vi "MGI RWA String To Anything.vi"(5 "Use Supplied":bool, 7 "Format String (%#_13g)":string="%#_13g", 8 "Error In":errorcluster, 9 "String":string, 10 "Type of Anything":variant, 11 "Read/Write Options":T1={"TS Fmt"="", "Int Fmt"="", "Delimiter"=","}) -> (0 "Error Out":errorcluster, 2 "Read Failures":string, 3 "Variant":variant)   [LabVIEW 2016]
doc: "Parse the specified String to populate the specified datatype. If string doesn't contain a field defined by datatype, then that field is set based on \"Use Supplied\". If \"Use Supplied\" is true, then the field is left as is, otherwise the field is set to default value.\n\nAuthored by Robert C. Mortensen\nsupport@mooregoodideas.com\nwww.mooregoodideas.com\n\nCopyright (c) 2010, Moore Good Ideas, Inc.\n\nAll rights reserved.\n\nRedistribution and use in source and binary forms, with or without modification, are permitted provided that the following conditions are met:\n\n * Redistributions of source code must retain the above copyright notice, this list of conditions and the following disclaimer.\n * Redistributions in binary form must reproduce the above copyright notice, this list of conditions and the following disclaimer in the documentation and/or other materials provided with the distribution.\n * Neither the name of Moore Good Ideas, Inc. nor the names of its contributors may be used to endorse or promote products derived from this software without specific prior written permission.\n\nTHIS SOFTWARE IS PROVIDED BY THE COPYRIGHT HOLDERS AND CONTRIBUTORS \"AS IS\" AND ANY EXPRESS OR IMPLIED WARRANTIES, INCLUDING, BUT NOT LIMITED TO, THE IMPLIED WARRANTIES OF MERCHANTABILITY AND FITNESS FOR A PARTICULAR PURPOSE ARE DISCLAIMED. IN NO EVENT SHALL THE COPYRIGHT OWNER OR CONTRIBUTORS BE LIABLE FOR ANY DIRECT, INDIRECT, INCIDENTAL, SPECIAL, EXEMPLARY, OR CONSEQUENTIAL DAMAGES (INCLUDING, BUT NOT LIMITED TO, PROCUREMENT OF SUBSTITUTE GOODS OR SERVICES; LOSS OF USE, DATA, OR PROFITS; OR BUSINESS INTERRUPTION) HOWEVER CAUSED AND ON ANY THEORY OF LIABILITY, WHETHER IN CONTRACT, STRICT LIABILITY, OR TORT (INCLUDING NEGLIGENCE OR OTHERWISE) ARISING IN ANY WAY OUT OF THE USE OF THIS SOFTWARE, EVEN IF ADVISED OF THE POSSIBILITY OF SUCH DAMAGE."
uses:
  <userlib>/_MGI/Read Write Anything/MGI RWA Options Cluster.ctl
  <userlib>/_MGI/Read Write Anything/MGI RWA Convertion Direction Enum.ctl
  <vilib>/Utility/VariantDataType/Type.ctl
  <userlib>/_MGI/String/MGI Scan From String/MGI Scan From String (CSG).vi
  <userlib>/_MGI/String/MGI Scan From String/MGI Scan From String (CDB).vi
  <userlib>/_MGI/String/MGI Scan From String/MGI Scan From String (CXT).vi
  <vilib>/Utility/VariantDataType/VariantType.lvlib
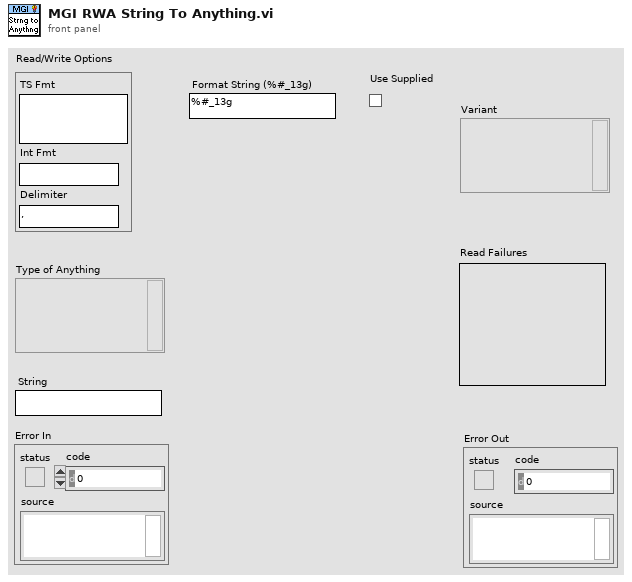
[diagram p1: front panel]
types:
  T1 = typedef "MGI RWA Options Cluster.ctl" = cluster{"TS Fmt":string, "Int Fmt":string, "Delimiter":string}
  T2 = typedef "MGI RWA Convertion Direction Enum.ctl" = enum16{"String->Anything", "Anything->String"}
  T3 = typedef "MGI RWA Tag Lookup Cluster.ctl" = cluster{"StrToSpecifiedText":variant, "Specified Data":variant, "Float Fmt":string, "Major Vers":i32, "Options":T1}
  T4 = typedef "VariantType.lvlib/Type.ctl" = enum8{"Invalid Type", "Void", "I8", "I16", "I32", "I64", "U8", "U16", "U32", "U64", "Single Float", "Double Float", "Extended Float", "Single Complex", "Double Complex", "Extended Complex", "Enum U8", "Enum U16", "Enum U32", "Enum U64", "Single Float With Unit", "Double Float With Unit", "Extended Float With Unit", "Single Complex with Unit", "Double Complex with Unit", "Extended Complex with Unit", "Boolean", "String", "Path", "Picture", "Tag", "Array", "Cluster", "Variant", "LV Variant", "Waveform", "Timestamp", "Digital Waveform", "Digital Data", "ExpressData", "Refnum", "External Data", "VI", "Poly VI", "LabVIEW Class Instance", "Fixed Point"}
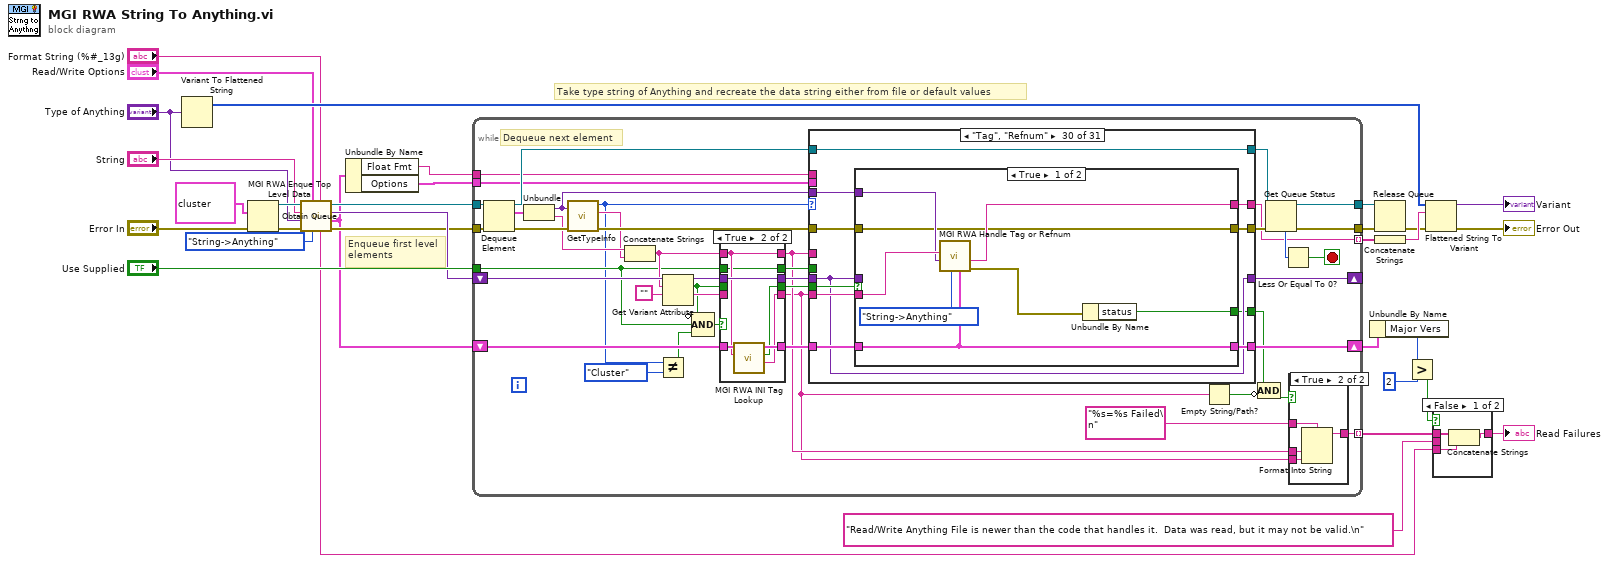
[diagram p0: block diagram]
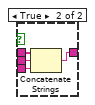
[diagram p2: hidden frame]
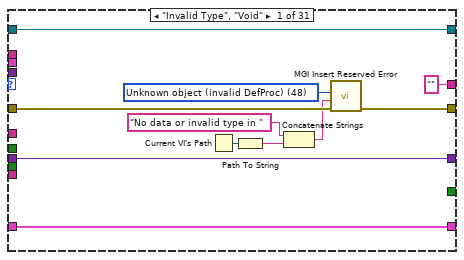
[diagram p5: hidden frame]
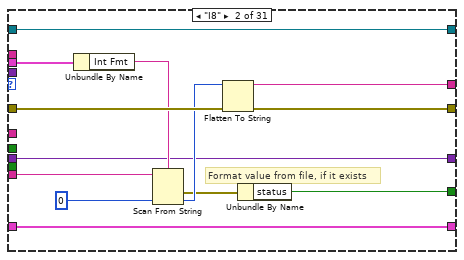
[diagram p6: hidden frame]
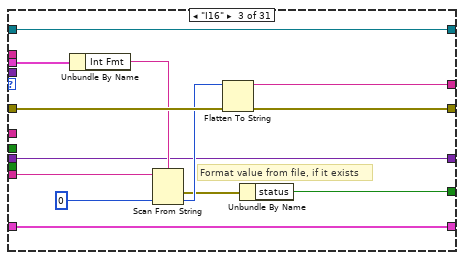
[diagram p7: hidden frame]
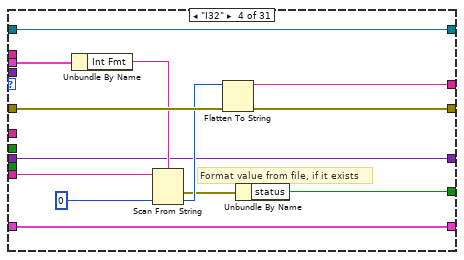
[diagram p8: hidden frame]
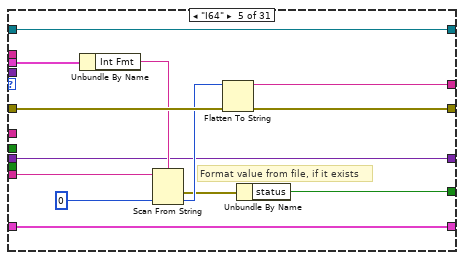
[diagram p9: hidden frame]
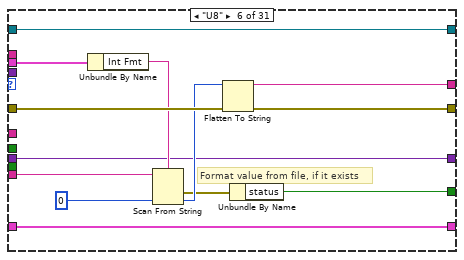
[diagram p10: hidden frame]
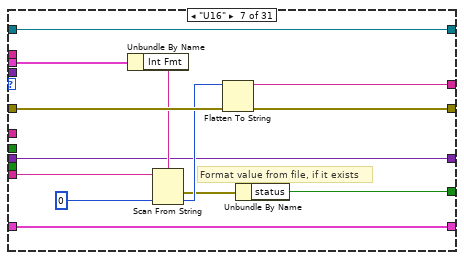
[diagram p11: hidden frame]
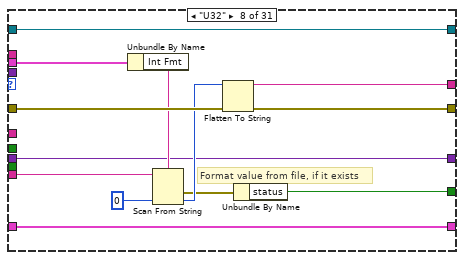
[diagram p12: hidden frame]
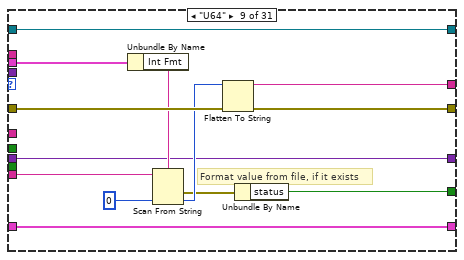
[diagram p13: hidden frame]
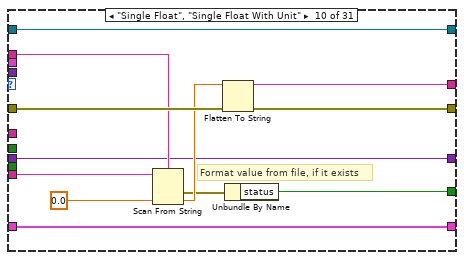
[diagram p14: hidden frame]
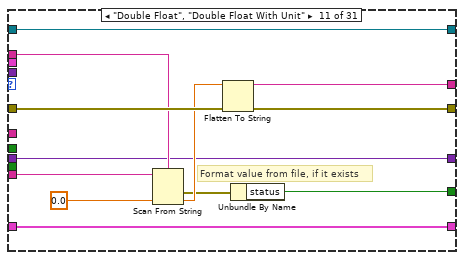
[diagram p15: hidden frame]
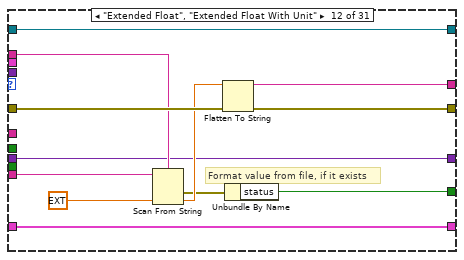
[diagram p16: hidden frame]
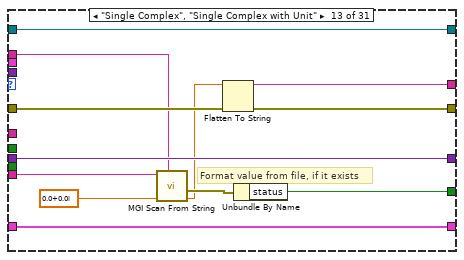
[diagram p17: hidden frame]
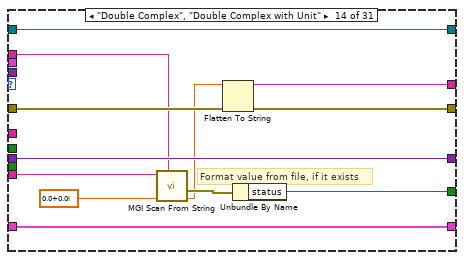
[diagram p18: hidden frame]
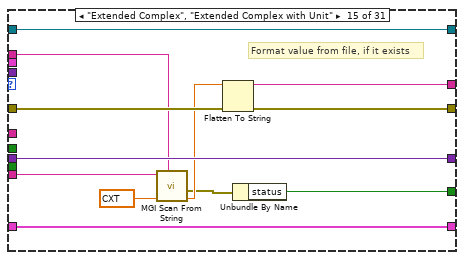
[diagram p19: hidden frame]
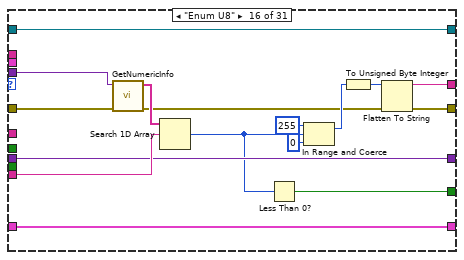
[diagram p20: hidden frame]
diagram:
  # "Enqueue first level\nelements"
  # "Take type string of Anything and recreate the data string either from file or default values"
  n1 = Variant To Flattened String(Variant="Type of Anything") -> (1:w25:i16[])  [unwired: 1 out]
  n2 = Obtain Queue(element data type=cluster{"Variant":variant, "Name":string} {"Variant"=variant, "Name"=""}, error in (no error)="Error In") -> (queue out=w23:refnum<queue>, error out=w17:errorcluster)  [unwired: 3 in, 1 out]
  n3 = call <userlib>:"MGI RWA Enque Top Level Data.vi"("Format String (%#_13g)"="Format String (%#_13g)", "Conversion"=MGI_RWA_Convertion_Direction_Enum."String->Anything", "Read/Write Options"="Read/Write Options", "Error In"=w17, "Anything"="Type of Anything", "Read String"="String", "Data Queue In"=w23) -> ("Error Out"=w20:errorcluster, "Read State"=w15:T3, "Tag to String"=w22:variant, "Data Queue Our"=w21:refnum<queue>, "Warnings"=w1:string)
  n4 = Unbundle By Name(w15) -> ("Float Fmt"=w13:string, "Options"=w11:T1)
  n5 = while {
    tunnel: w20 -> [w74]
    tunnel: [w40] -> w28
    tunnel: [w61] -> w27 mode=indexing
    tunnel: w21 -> [w71]
    tunnel: [w66] -> w30
    tunnel: w11 -> [w42]
    tunnel: w13 -> [w41]
    shift-right: [w47] -> w10
    shift-left: w15 -> [w51]
    shift-right: [w46] -> _
    shift-left: w22 -> [w59]
    tunnel: "Use Supplied" -> [w50]
    tunnel: [w33] -> w6 mode=indexing
    stop <- w67 stop-if-true
    # "Dequeue next element"
    n6 = Dequeue Element(queue=w71, error in (no error)=w74) -> (queue out=w72:refnum<queue>, element=w65:cluster{"Variant":variant, "Name":string}, error out=w73:errorcluster)  [unwired: 1 in, 1 out]
    n7 = Unbundle(w65) -> ("Variant"=w63:variant, "Name"=w64:string)
    n8 = call <vilib>:"GetTypeInfo.vi"("error in (no error)"=w73, "Variant"=w63) -> ("error out"=w75:errorcluster, "Name"=w62:string, "Type Enum"=w45:T4)  [unwired: 5 in, 2 out]
    n9 = Concatenate Strings(w64, w62) -> (w55:string)
    n10 = Not Equal?(x=w45, y=Type."Cluster") -> (x != y?=w44:bool)
    n11 = Get Variant Attribute(Variant=w59, name=w55, default value (empty Variant)="") -> (duplicate Variant=w54:variant, found=w57:bool, value=w58:string)  [unwired: 1 in, 1 out]
    n12 = Compound Arithmetic op=AND(invert w57, w50, w44) -> (w56:bool)
    n13 = case shown="True" w56 {
      tunnel: w58 -> [w82 _]
      tunnel: w57 -> [w83 _]
      tunnel: w55 -> [w84 w87]
      tunnel: w54 -> [w85 w91]
      tunnel: [w85 w91] -> w53
      tunnel: [w84 w87] -> w36
      tunnel: [w83 w89] -> w52
      tunnel: [w82 w88] -> w35
      tunnel: w51 -> [w81 w92]
      tunnel: [w81 w90] -> w48
      tunnel: w50 -> [w80 w86]
      tunnel: [w80 w86] -> w49
      frame False {
      }
      frame True {
        n14 = call <userlib>:"MGI RWA INI Tag Lookup.vi"("String"=w87, "State In"=w92) -> ("INI Text"=w88:string, "Text Found?"=w89:bool, "State Out"=w90:T3)  [unwired: 7 in]
      }
    }
    n15 = case shown="\"Tag\", \"Refnum\"" w45 {
      tunnel: [w97 w116 w129 w142 w155 w168 w181 w194 w207 w219 w231 w243 w255 w267 w279 w295 w311 w327 w343 w353 w361 w369 w377 w398 w426 w459 w505 w533 w565 w580 w601] -> w70
      tunnel: w75 -> [w98 w115 w128 w141 w154 w167 w180 w193 w206 w218 w230 w242 w254 w266 w278 w294 w310 w326 w342 w352 w360 w368 w383 w397 w425 w458 w504 w532 w568 w579 w600]
      tunnel: w36 -> [_ _ _ _ _ _ _ _ _ _ _ _ _ _ _ _ _ _ _ _ _ _ w370 _ _ _ _ _ w562 _ _]
      tunnel: ["" ("data string") w114 w127 w140 w153 w166 w179 w192 w205 w217 w229 w241 w253 w265 w277 w293 w309 w325 w341 w351 w359 w367 "" w396 w424 w457 w503 w531 w557 w578 w599] -> w61
      tunnel: w63 -> [_ _ _ _ _ _ _ _ _ _ _ _ _ _ _ w292 w308 w324 w340 _ _ _ w382 _ _ _ _ _ w567 w571 _]
      tunnel: w72 -> [w99 w113 w126 w139 w152 w165 w178 w191 w204 w216 w228 w240 w252 w264 w276 w291 w307 w323 w339 w350 w358 w366 w378 w395 w423 w456 w502 w530 w569 w577 w598]
      tunnel: [w99 w113 w126 w139 w152 w165 w178 w191 w204 w216 w228 w240 w252 w264 w276 w291 w307 w323 w339 w350 w358 w366 w376 w395 w423 w456 w502 w530 w564 w577 w598] -> w69
      tunnel: w53 -> [w94 w108 w121 w134 w147 w160 w173 w186 w200 w211 w223 w235 w251 w263 w275 w283 w299 w316 w331 w345 w356 w363 w372 w393 w420 w449 w499 w527 w561 w572 w595]
      tunnel: w42 -> [_ w106 w119 w132 w145 w158 w171 w184 w197 _ _ _ _ _ _ _ _ _ _ _ _ _ _ _ _ _ _ _ w556 _ _]
      tunnel: w41 -> [_ _ _ _ _ _ _ _ _ w213 w225 w237 w246 w259 w270 _ _ _ _ _ _ _ _ _ _ _ _ _ w555 _ _]
      tunnel: [w94 w108 w121 w134 w147 w160 w173 w186 w200 w211 w223 w235 w251 w263 w275 w283 w299 w316 w331 w345 w356 w363 w372 w393 w420 w449 w499 w527 w558 w572 w595] -> w46
      tunnel: w35 -> [_ w109 w122 w135 w148 w161 w174 w187 w199 w212 w224 w236 w245 w256 w271 w284 w300 w317 w332 w346 w357 w364 _ w394 w422 w450 w500 w528 w566 w575 w596]
      tunnel: w52 -> [_ _ _ _ _ _ _ _ _ _ _ _ _ _ _ _ _ _ _ _ _ _ _ w392 w421 w451 w501 w529 _ w576 w597]
      tunnel: w49 -> [_ _ _ _ _ _ _ _ _ _ _ _ _ _ _ _ _ _ _ _ _ _ _ _ _ _ _ _ w563 _ _]
      tunnel: w48 -> [w93 w107 w120 w133 w146 w159 w172 w185 w198 w210 w222 w234 w250 w262 w274 w282 w298 w315 w330 w344 w355 w362 w371 w391 w419 w448 w498 w526 w560 w574 w594]
      tunnel: [w93 w107 w120 w133 w146 w159 w172 w185 w198 w210 w222 w234 w250 w262 w274 w282 w298 w315 w330 w344 w355 w362 w371 w391 w419 w448 w498 w526 w559 w573 w594] -> w47
      tunnel: [_ w104 w117 w130 w143 w156 w169 w182 w195 w208 w220 w232 w249 w261 w273 w280 w296 w312 w328 _ _ _ _ _ _ w447 _ _ w554 w570 _] -> w39
      frame "Invalid Type", "Void" {
        w95 = u16 48 items=["No error", "Argument error", "Memory is full", "Out of zone", "End of file", "File already open", "Generic file I/O error", "File not found", "File permission error", "Disk is full", "Duplicate path", "Too many files open", "System feature not enabled", "Resource file not found", "Cannot add resource", "Resource not found", "Image not found", "Image memory error", "Pen does not exist", "Config type invalid", "Config token not found", "Config parse error", "Config memory error", "Bad external code format", "Bad external code offset", "External code not present", "Null window", "Destroy window error", "Null menu", "Print aborted", "Bad print record", "Print driver error", "Windows error during printing", "Memory error during printing", "Print dialog error", "Generic print error", "Invalid device refnum", "Device not found", "Device parameter error", "Device unit error", "Cannot open device", "Device call aborted", "Generic error", "Cancelled by user", "Object ID too low", "Object ID too high", "Object not in heap", "Unknown heap", "Unknown object (invalid DefProc)", "Unknown object (DefProc not in table)", "Message out of range", "Invalid (null) method", "Unknown message", "Manager call not supported", "Bad address", "Network operation in progress", "Network operation timed out", "Connection is busy", "Network attribute not supported", "Network error", "Address in use", "System out of memory", "Connection aborted", "Connection refused", "Not connected", "Already connected", "Connection closed", "Initialization error (interapplication manager)", "Bad occurrence", "Wait on unbound occurrence handler", "Occurrence queue overflow", "Datalog type conflict", "Unused", "Unrecognized type (interapplication manager)", "Memory corrupt", "Failed to make temporary DLL", "Old CIN version", "Drag socket not found", "Failed to load drop-object", "Failed to register OLE object", "Failed to release OLE object", "Format specifier type mismatch", "Unknown format specifier", "Too few format specifiers", "Too many format specifiers", "Scan failed", "Newer CIN version", "OLE Convert", "Runtime menu error", "Password tampered", "Unknown error code"] ("Reserved Error Code")
        n16 = Current VI's Path() -> (path=w101:path)
        n17 = Path To String(path=w101) -> (string=w100:string)
        n18 = Concatenate Strings("No data or invalid type in " ("string"), w100) -> (w96:string)
        n19 = call <userlib>:"MGI Insert Reserved Error.vi"("Error In"=w98, "Error Description"=w96, "Reserved Error Code (Generic error)"=w95) -> ("Error Out"=w97:errorcluster)  [unwired: 8 in]
      }
      frame "I8" {
        # "Format value from file, if it exists"
        n20 = Unbundle By Name(w106) -> ("Int Fmt"=w111:string)
        n21 = Scan From String(format string=w111, input string=w109, default 1=i8 0 ("default (0 I32)")) -> (error out=w105:errorcluster, output 1=w110:i8)  [unwired: 2 in, 2 out]
        n22 = Flatten To String(anything=w110, error in (no error)=w115) -> (data string=w114:string, error out=w116:errorcluster)  [unwired: 2 in, 1 out]
        n23 = Unbundle By Name(w105) -> ("status"=w104:bool)
      }
      frame "I16" {
        # "Format value from file, if it exists"
        n24 = Unbundle By Name(w119) -> ("Int Fmt"=w124:string)
        n25 = Scan From String(format string=w124, input string=w122, default 1=i16 0 ("default (0 I32)")) -> (error out=w118:errorcluster, output 1=w123:i16)  [unwired: 2 in, 2 out]
        n26 = Flatten To String(anything=w123, error in (no error)=w128) -> (data string=w127:string, error out=w129:errorcluster)  [unwired: 2 in, 1 out]
        n27 = Unbundle By Name(w118) -> ("status"=w117:bool)
      }
      frame "I32" {
        # "Format value from file, if it exists"
        n28 = Unbundle By Name(w132) -> ("Int Fmt"=w137:string)
        n29 = Scan From String(format string=w137, input string=w135, default 1=0 ("default (0 I32)")) -> (error out=w131:errorcluster, output 1=w136:i32)  [unwired: 2 in, 2 out]
        n30 = Flatten To String(anything=w136, error in (no error)=w141) -> (data string=w140:string, error out=w142:errorcluster)  [unwired: 2 in, 1 out]
        n31 = Unbundle By Name(w131) -> ("status"=w130:bool)
      }
      frame "I64" {
        # "Format value from file, if it exists"
        n32 = Unbundle By Name(w145) -> ("Int Fmt"=w150:string)
        n33 = Scan From String(format string=w150, input string=w148, default 1=i64 0 ("default (0 I32)")) -> (error out=w144:errorcluster, output 1=w149:i64)  [unwired: 2 in, 2 out]
        n34 = Flatten To String(anything=w149, error in (no error)=w154) -> (data string=w153:string, error out=w155:errorcluster)  [unwired: 2 in, 1 out]
        n35 = Unbundle By Name(w144) -> ("status"=w143:bool)
      }
      frame "U8" {
        # "Format value from file, if it exists"
        n36 = Unbundle By Name(w158) -> ("Int Fmt"=w163:string)
        n37 = Scan From String(format string=w163, input string=w161, default 1=u8 0 ("default (0 I32)")) -> (error out=w157:errorcluster, output 1=w162:u8)  [unwired: 2 in, 2 out]
        n38 = Flatten To String(anything=w162, error in (no error)=w167) -> (data string=w166:string, error out=w168:errorcluster)  [unwired: 2 in, 1 out]
        n39 = Unbundle By Name(w157) -> ("status"=w156:bool)
      }
      frame "U16" {
        # "Format value from file, if it exists"
        n40 = Unbundle By Name(w171) -> ("Int Fmt"=w176:string)
        n41 = Scan From String(format string=w176, input string=w174, default 1=u16 0 ("default (0 I32)")) -> (error out=w170:errorcluster, output 1=w175:u16)  [unwired: 2 in, 2 out]
        n42 = Flatten To String(anything=w175, error in (no error)=w180) -> (data string=w179:string, error out=w181:errorcluster)  [unwired: 2 in, 1 out]
        n43 = Unbundle By Name(w170) -> ("status"=w169:bool)
      }
      frame "U32" {
        # "Format value from file, if it exists"
        n44 = Unbundle By Name(w184) -> ("Int Fmt"=w189:string)
        n45 = Scan From String(format string=w189, input string=w187, default 1=u32 0 ("default (0 I32)")) -> (error out=w183:errorcluster, output 1=w188:u32)  [unwired: 2 in, 2 out]
        n46 = Flatten To String(anything=w188, error in (no error)=w193) -> (data string=w192:string, error out=w194:errorcluster)  [unwired: 2 in, 1 out]
        n47 = Unbundle By Name(w183) -> ("status"=w182:bool)
      }
      frame "U64" {
        # "Format value from file, if it exists"
        n48 = Unbundle By Name(w197) -> ("Int Fmt"=w202:string)
        n49 = Scan From String(format string=w202, input string=w199, default 1=u64 0 ("default (0 I32)")) -> (error out=w196:errorcluster, output 1=w201:u64)  [unwired: 2 in, 2 out]
        n50 = Flatten To String(anything=w201, error in (no error)=w206) -> (data string=w205:string, error out=w207:errorcluster)  [unwired: 2 in, 1 out]
        n51 = Unbundle By Name(w196) -> ("status"=w195:bool)
      }
      frame "Single Float", "Single Float With Unit" {
        # "Format value from file, if it exists"
        n52 = Scan From String(format string=w213, input string=w212, default 1=sgl 0.0 ("default (0 I32)")) -> (error out=w209:errorcluster, output 1=w214:sgl)  [unwired: 2 in, 2 out]
        n53 = Flatten To String(anything=w214, error in (no error)=w218) -> (data string=w217:string, error out=w219:errorcluster)  [unwired: 2 in, 1 out]
        n54 = Unbundle By Name(w209) -> ("status"=w208:bool)
      }
      frame "Double Float", "Double Float With Unit" {
        # "Format value from file, if it exists"
        n55 = Scan From String(format string=w225, input string=w224, default 1=0.0 ("default (0 I32)")) -> (error out=w221:errorcluster, output 1=w226:dbl)  [unwired: 2 in, 2 out]
        n56 = Flatten To String(anything=w226, error in (no error)=w230) -> (data string=w229:string, error out=w231:errorcluster)  [unwired: 2 in, 1 out]
        n57 = Unbundle By Name(w221) -> ("status"=w220:bool)
      }
      frame "Extended Float", "Extended Float With Unit" {
        # "Format value from file, if it exists"
        n58 = Scan From String(format string=w237, input string=w236, default 1=ext 0.0 ("default (0 I32)")) -> (error out=w233:errorcluster, output 1=w238:ext)  [unwired: 2 in, 2 out]
        n59 = Flatten To String(anything=w238, error in (no error)=w242) -> (data string=w241:string, error out=w243:errorcluster)  [unwired: 2 in, 1 out]
        n60 = Unbundle By Name(w233) -> ("status"=w232:bool)
      }
      frame "Single Complex", "Single Complex with Unit" {
        # "Format value from file, if it exists"
        n61 = call-poly <userlib>:"MGI Scan From String.vi"("format string"=w246, "Default CSG[]"=csg 0.0+0.0i ("default (0 I32)"), "String In"=w245) -> ("CSG[] Out"=w247:csg, "error out"=w248:errorcluster)  [unwired: 5 in, 2 out]
        n62 = Flatten To String(anything=w247, error in (no error)=w254) -> (data string=w253:string, error out=w255:errorcluster)  [unwired: 2 in, 1 out]
        n63 = Unbundle By Name(w248) -> ("status"=w249:bool)
      }
      frame "Double Complex", "Double Complex with Unit" {
        # "Format value from file, if it exists"
        n64 = call-poly <userlib>:"MGI Scan From String.vi"("format string"=w259, "Default CXT[]"=cdb 0.0+0.0i ("default (0 I32)"), "String In"=w256) -> ("CXT[] Out"=w257:cdb, "error out"=w258:errorcluster)  [unwired: 5 in, 2 out]
        n65 = Flatten To String(anything=w257, error in (no error)=w266) -> (data string=w265:string, error out=w267:errorcluster)  [unwired: 2 in, 1 out]
        n66 = Unbundle By Name(w258) -> ("status"=w261:bool)
      }
      frame "Extended Complex", "Extended Complex with Unit" {
        # "Format value from file, if it exists"
        n67 = call-poly <userlib>:"MGI Scan From String.vi"("format string"=w270, "Default CXT[]"=cxt 0.0+0.0i ("default (0 I32)"), "String In"=w271) -> ("CXT[] Out"=w269:cxt, "error out"=w268:errorcluster)  [unwired: 5 in, 2 out]
        n68 = Flatten To String(anything=w269, error in (no error)=w278) -> (data string=w277:string, error out=w279:errorcluster)  [unwired: 2 in, 1 out]
        n69 = Unbundle By Name(w268) -> ("status"=w273:bool)
      }
      frame "Enum U8" {
        n70 = call <vilib>:"GetNumericInfo.vi"("error in (no error)"=w294, "Variant"=w292) -> ("error out"=w285:errorcluster, "EnumNames"=w290:string[])  [unwired: 6 in, 2 out]
        n71 = Search 1D Array(1D array=w290, element=w284) -> (index of element=w281:i32)  [unwired: 1 in]
        n72 = Less Than 0?(x=w281) -> (x < 0?=w280:bool)
        n73 = In Range and Coerce(upper limit=255, x=w281, lower limit=0) -> (coerced(x)=w288:i32)  [unwired: 1 out]
        n74 = To Unsigned Byte Integer(number=w288) -> (unsigned 8bit integer=w289:u8)
        n75 = Flatten To String(anything=w289, error in (no error)=w285) -> (data string=w293:string, error out=w295:errorcluster)  [unwired: 2 in, 1 out]
      }
      frame "Enum U16" {
        n76 = call <vilib>:"GetNumericInfo.vi"("error in (no error)"=w310, "Variant"=w308) -> ("error out"=w304:errorcluster, "EnumNames"=w306:string[])  [unwired: 6 in, 2 out]
        n77 = Search 1D Array(1D array=w306, element=w300) -> (index of element=w297:i32)  [unwired: 1 in]
        n78 = In Range and Coerce(upper limit=65535, x=w297, lower limit=0) -> (coerced(x)=w302:i32)  [unwired: 1 out]
        n79 = Less Than 0?(x=w297) -> (x < 0?=w296:bool)
        n80 = To Unsigned Word Integer(number=w302) -> (unsigned 16bit integer=w301:u16)
        n81 = Flatten To String(anything=w301, error in (no error)=w304) -> (data string=w309:string, error out=w311:errorcluster)  [unwired: 2 in, 1 out]
      }
      frame "Enum U32" {
        n82 = call <vilib>:"GetNumericInfo.vi"("error in (no error)"=w326, "Variant"=w324) -> ("error out"=w320:errorcluster, "EnumNames"=w322:string[])  [unwired: 6 in, 2 out]
        n83 = Search 1D Array(1D array=w322, element=w317) -> (index of element=w313:i32)  [unwired: 1 in]
        n84 = Less Than 0?(x=w313) -> (x < 0?=w312:bool)
        n85 = In Range and Coerce(upper limit=2147483647, x=w313, lower limit=0) -> (coerced(x)=w319:i32)  [unwired: 1 out]
        n86 = To Unsigned Long Integer(number=w319) -> (unsigned 32bit integer=w318:u32)
        n87 = Flatten To String(anything=w318, error in (no error)=w320) -> (data string=w325:string, error out=w327:errorcluster)  [unwired: 2 in, 1 out]
      }
      frame "Enum U64" {
        n88 = call <vilib>:"GetNumericInfo.vi"("error in (no error)"=w342, "Variant"=w340) -> ("error out"=w336:errorcluster, "EnumNames"=w338:string[])  [unwired: 6 in, 2 out]
        n89 = Search 1D Array(1D array=w338, element=w332) -> (index of element=w329:i32)  [unwired: 1 in]
        n90 = Less Than 0?(x=w329) -> (x < 0?=w328:bool)
        n91 = In Range and Coerce(upper limit=2147483647, x=w329, lower limit=0) -> (coerced(x)=w333:i32)  [unwired: 1 out]
        n92 = To Unsigned Quad Integer(1:w333) -> (0:w334:u64)
        n93 = Flatten To String(anything=w334, error in (no error)=w336) -> (data string=w341:string, error out=w343:errorcluster)  [unwired: 2 in, 1 out]
      }
      frame "Boolean" {
        n94 = call <vilib>:"Trim Whitespace.vi"("string"=w346) -> ("trimmed string"=w348:string)  [unwired: 1 in]
        n95 = To Upper Case(1:w348) -> (0:w347:string)
        n96 = case shown="Default" w347 {
          tunnel: [_ TRUE] -> w349
          frame Default {
          }
          frame "1", "ON", "TRUE", "YES" {
          }
        }
        n97 = Flatten To String(anything=w349, error in (no error)=w352) -> (data string=w351:string, error out=w353:errorcluster)  [unwired: 2 in, 1 out]
      }
      frame "String" {
        n98 = Flatten To String(anything=w357, error in (no error)=w360) -> (data string=w359:string, error out=w361:errorcluster)  [unwired: 2 in, 1 out]
      }
      frame "Path" {
        n99 = String To Path(string=w364) -> (path=w365:path)
        n100 = Flatten To String(anything=w365, error in (no error)=w368) -> (data string=w367:string, error out=w369:errorcluster)  [unwired: 2 in, 1 out]
      }
      frame "Cluster" {
        # "Enqueue cluster elements"
        n101 = call <vilib>:"GetClusterInfo.vi"("error in (no error)"=w383, "Variant"=w382) -> ("error out"=w379:errorcluster, "Cluster Elements"=w381:variant[])  [unwired: 8 in]
        n102 = Concatenate Strings(w370, "." ("string")) -> (w373:string)
        n103 = Reverse 1D Array(array=w381) -> (reversed array=w380:variant[])
        n104 = for {
          tunnel: w378 -> [w390]
          tunnel: w379 -> [w389]
          tunnel: [w388] -> w377
          tunnel: [w387] -> w376
          tunnel: w380 -> [w386] mode=indexing
          tunnel: w373 -> [w384]
          n105 = Bundle("ArrayElt"=w386, w384) -> (w385:cluster{"ArrayElt":variant, string})  [unwired: 1 in]
          n106 = Enqueue Element At Opposite End(queue=w390, element=w385, error in (no error)=w389) -> (queue out=w387:refnum<queue>, error out=w388:errorcluster)  [unwired: 1 in, 1 out]
        }
      }
      frame "Variant", "LV Variant" {
        n107 = case shown="True" w392 {
          tunnel: w394 -> [w399 _]
          tunnel: [w407 w416] -> w398
          tunnel: w397 -> [w407 w417]
          tunnel: [w405 w418] -> w396
          frame True {
            n108 = String Subset(string=w399, offset (0)=2) -> (substring=w404:string)  [unwired: 1 in]
            n109 = String Length(string=w404) -> (length=w402:i32)
            n110 = Multiply(x=0.5, y=w402) -> (x*y=w401:dbl)
            n111 = for {
              N: w401 -> [_]
              tunnel: w404 -> [w411]
              tunnel: [w413] -> w403 mode=indexing
              i -> [w410]
              w409 = 2 ("length (rest)")
              n112 = Multiply(x=w410, y=w409) -> (x*y=w408:i32)
              n113 = String Subset(string=w411, offset (0)=w408, length (rest)=w409) -> (substring=w412:string)
              n114 = Hexadecimal String To Number(string=w412, default (0uL)=u8 0 ("default (0 U32)")) -> (number=w413:u8)  [unwired: 1 in, 1 out]
            }
            n115 = Byte Array To String(unsigned byte array=w403) -> (string=w405:string)
          }
          frame False {
            w415 = variant  # Variant
            n116 = Flatten To String(anything=w415, error in (no error)=w417) -> (data string=w418:string, error out=w416:errorcluster)  [unwired: 2 in, 1 out]
          }
        }
      }
      frame "Waveform" {
        n117 = case shown="True" w421 {
          tunnel: w422 -> [w427 _]
          tunnel: [w435 w445] -> w426
          tunnel: w425 -> [w435 w444]
          tunnel: [w433 w446] -> w424
          frame True {
            n118 = String Subset(string=w427, offset (0)=2) -> (substring=w432:string)  [unwired: 1 in]
            n119 = String Length(string=w432) -> (length=w430:i32)
            n120 = Multiply(x=0.5, y=w430) -> (x*y=w429:dbl)
            n121 = for {
              N: w429 -> [_]
              tunnel: w432 -> [w439]
              tunnel: [w441] -> w431 mode=indexing
              i -> [w438]
              w437 = 2 ("length (rest)")
              n122 = Multiply(x=w438, y=w437) -> (x*y=w436:i32)
              n123 = String Subset(string=w439, offset (0)=w436, length (rest)=w437) -> (substring=w440:string)
              n124 = Hexadecimal String To Number(string=w440, default (0uL)=u8 0 ("default (0 U32)")) -> (number=w441:u8)  [unwired: 1 in, 1 out]
            }
            n125 = Byte Array To String(unsigned byte array=w431) -> (string=w433:string)
          }
          frame False {
            n126 = Flatten To String(anything=waveform(dbl) {"t0"=timestamp(0 s since 1904-01-01), "dt"=0.0, "Y"=[]} ("Waveform 2"), error in (no error)=w444) -> (data string=w446:string, error out=w445:errorcluster)  [unwired: 2 in, 1 out]
          }
        }
      }
      frame "Timestamp" {
        n127 = Unbundle By Name(w448) -> ("Options.TS Fmt"=w455:string)
        n128 = Match First String(2:string[] ["0x"] ("string array"), 3:w450) -> (0:w453:i32, 1:w452:string)
        n129 = case shown="True" w451 {
          tunnel: [w462 w496] -> w459
          tunnel: w458 -> [w463 w495]
          tunnel: [w466 w497] -> w457
          tunnel: w455 -> [w465 _]
          tunnel: w453 -> [w461 _]
          tunnel: w452 -> [w464 _]
          tunnel: [w460 _] -> w447
          frame True {
            n130 = case shown="0.." w461 {
              tunnel: [w469 w491] -> w466
              tunnel: w465 -> [_ w487]
              tunnel: w464 -> [w471 w490]
              tunnel: w463 -> [w470 w489]
              tunnel: [w470 w488] -> w462
              tunnel: [FALSE ("status") w482] -> w460
              frame 0.. {
                n131 = String Length(string=w471) -> (length=w472:i32)
                n132 = Quotient & Remainder(x=w472, y=2) -> (floor(x/y)=w474:i32)  [unwired: 1 out]
                n133 = for {
                  N: w474 -> [_]
                  tunnel: w471 -> [w478]
                  tunnel: [w480] -> w468 mode=indexing
                  i -> [w477]
                  w476 = 2 ("length (rest)")
                  n134 = Multiply(x=w477, y=w476) -> (x*y=w475:i32)
                  n135 = String Subset(string=w478, offset (0)=w475, length (rest)=w476) -> (substring=w479:string)
                  n136 = Hexadecimal String To Number(string=w479, default (0uL)=u8 0 ("default (0 U32)")) -> (number=w480:u8)  [unwired: 1 in, 1 out]
                }
                n137 = Byte Array To String(unsigned byte array=w468) -> (string=w469:string)
              }
              frame ..-1 {
                n138 = Concatenate Strings("%<" ("string"), w487, ">T" ("string")) -> (w486:string)
                n139 = Scan From String(format string=w486, input string=w490, default 1=timestamp(0 s since 1904-01-01)) -> (error out=w483:errorcluster, output 1=w492:timestamp)  [unwired: 2 in, 2 out]
                n140 = Unbundle By Name(w483) -> ("status"=w482:bool)
                n141 = Flatten To String(anything=w492, error in (no error)=w489) -> (data string=w491:string, error out=w488:errorcluster)  [unwired: 2 in, 1 out]
              }
            }
          }
          frame False {
            n142 = Flatten To String(anything=timestamp(0 s since 1904-01-01), error in (no error)=w495) -> (data string=w497:string, error out=w496:errorcluster)  [unwired: 2 in, 1 out]
          }
        }
      }
      frame "Digital Waveform" {
        n143 = case shown="True" w501 {
          tunnel: w500 -> [w506 _]
          tunnel: [w514 w524] -> w505
          tunnel: w504 -> [w514 w523]
          tunnel: [w512 w525] -> w503
          frame True {
            n144 = String Subset(string=w506, offset (0)=2) -> (substring=w511:string)  [unwired: 1 in]
            n145 = String Length(string=w511) -> (length=w509:i32)
            n146 = Multiply(x=0.5, y=w509) -> (x*y=w508:dbl)
            n147 = for {
              N: w508 -> [_]
              tunnel: w511 -> [w518]
              tunnel: [w520] -> w510 mode=indexing
              i -> [w517]
              w516 = 2 ("length (rest)")
              n148 = Multiply(x=w517, y=w516) -> (x*y=w515:i32)
              n149 = String Subset(string=w518, offset (0)=w515, length (rest)=w516) -> (substring=w519:string)
              n150 = Hexadecimal String To Number(string=w519, default (0uL)=u8 0 ("default (0 U32)")) -> (number=w520:u8)  [unwired: 1 in, 1 out]
            }
            n151 = Byte Array To String(unsigned byte array=w510) -> (string=w512:string)
          }
          frame False {
            n152 = call <vilib>:"DWDT Empty Digital.vi"() -> ("digital waveform out"=w522:digitalwaveform)  [unwired: 5 in]
            n153 = Flatten To String(anything=w522, error in (no error)=w523) -> (data string=w525:string, error out=w524:errorcluster)  [unwired: 2 in, 1 out]
          }
        }
      }
      frame "Digital Data" {
        n154 = case shown="True" w529 {
          tunnel: w528 -> [w534 _]
          tunnel: [w542 w552] -> w533
          tunnel: w532 -> [w542 w551]
          tunnel: [w540 w553] -> w531
          frame True {
            n155 = String Subset(string=w534, offset (0)=2) -> (substring=w539:string)  [unwired: 1 in]
            n156 = String Length(string=w539) -> (length=w537:i32)
            n157 = Multiply(x=0.5, y=w537) -> (x*y=w536:dbl)
            n158 = for {
              N: w536 -> [_]
              tunnel: w539 -> [w546]
              tunnel: [w548] -> w538 mode=indexing
              i -> [w545]
              w544 = 2 ("length (rest)")
              n159 = Multiply(x=w545, y=w544) -> (x*y=w543:i32)
              n160 = String Subset(string=w546, offset (0)=w543, length (rest)=w544) -> (substring=w547:string)
              n161 = Hexadecimal String To Number(string=w547, default (0uL)=u8 0 ("default (0 U32)")) -> (number=w548:u8)  [unwired: 1 in, 1 out]
            }
            n162 = Byte Array To String(unsigned byte array=w538) -> (string=w540:string)
          }
          frame False {
            n163 = call <vilib>:"DTbl Empty Digital.vi"() -> ("digital data"=w550:digitaldata)  [unwired: 5 in]
            n164 = Flatten To String(anything=w550, error in (no error)=w551) -> (data string=w553:string, error out=w552:errorcluster)  [unwired: 2 in, 1 out]
          }
        }
      }
      frame "Array" {
        n165 = call <userlib>:"MGI RWA Unprocess Array Elements.vi"("Queue In"=w569, "Value"=w566, "Read/Write Options"=w556, "Format String (%#_13g)"=w555, "Array Variant"=w567, "Name In"=w562, "Str to INI in"=w561, "Error In"=w568, "Use Specified?"=w563, "State In"=w560) -> ("Queue Out"=w564:refnum<queue>, "Scan Failed?"=w554:bool, "Data Out"=w557:string, "Str to INI out"=w558:variant, "State Out"=w559:T3, "Error Out"=w565:errorcluster)
      }
      frame "Tag", "Refnum" {
        n166 = case shown="True" w576 {
          tunnel: w575 -> [w586 _]
          tunnel: [w583 w591] -> w580
          tunnel: w579 -> [w583 w592]
          tunnel: [w588 w593] -> w578
          tunnel: w574 -> [w587 w589]
          tunnel: [w587 w589] -> w573
          tunnel: w572 -> [_ _]
          tunnel: w571 -> [w584 _]
          tunnel: [w581 _] -> w570
          frame True {
            n167 = call <userlib>:"MGI RWA Handle Tag or Refnum.vi"("Read State In"=w587, "Conversion"=MGI_RWA_Convertion_Direction_Enum."String->Anything", "Anything"=w584, "Read String"=w586) -> ("Error Out"=w582:errorcluster, "String"=w588:string)  [unwired: 6 in]
            n168 = Unbundle By Name(w582) -> ("status"=w581:bool)
          }
          frame False {
            n169 = Flatten To String(anything="", error in (no error)=w592) -> (data string=w593:string, error out=w591:errorcluster)  [unwired: 2 in, 1 out]
          }
        }
      }
      frame Default {
        n170 = case shown="True" w597 {
          tunnel: w596 -> [w602 _]
          tunnel: [w610 w619] -> w601
          tunnel: w600 -> [w610 w620]
          tunnel: [w608 w621] -> w599
          frame True {
            n171 = String Subset(string=w602, offset (0)=2) -> (substring=w607:string)  [unwired: 1 in]
            n172 = String Length(string=w607) -> (length=w605:i32)
            n173 = Multiply(x=0.5, y=w605) -> (x*y=w603:dbl)
            n174 = for {
              N: w603 -> [_]
              tunnel: w607 -> [w614]
              tunnel: [w616] -> w606 mode=indexing
              i -> [w613]
              w612 = 2 ("length (rest)")
              n175 = Multiply(x=w613, y=w612) -> (x*y=w611:i32)
              n176 = String Subset(string=w614, offset (0)=w611, length (rest)=w612) -> (substring=w615:string)
              n177 = Hexadecimal String To Number(string=w615, default (0uL)=u8 0 ("default (0 U32)")) -> (number=w616:u8)  [unwired: 1 in, 1 out]
            }
            n178 = Byte Array To String(unsigned byte array=w606) -> (string=w608:string)
          }
          frame False {
            n179 = Flatten To String(anything="", error in (no error)=w620) -> (data string=w621:string, error out=w619:errorcluster)  [unwired: 2 in, 1 out]
          }
        }
      }
    }
    n180 = Empty String/Path?(string/path=w35) -> (empty?=w38:bool)
    n181 = Compound Arithmetic op=AND(w39, invert w38) -> (w37:bool)
    n182 = Get Queue Status(queue=w69, error in (no error)=w70) -> (queue out=w66:refnum<queue>, error out=w40:errorcluster, # elements in queue=w68:i32)  [unwired: 1 in, 5 out]
    n183 = Less Or Equal To 0?(x=w68) -> (x <= 0?=w67:bool)
    n184 = case shown="True" w37 {
      tunnel: w36 -> [_ w79]
      tunnel: w35 -> [_ w78]
      tunnel: "%s=%s Failed\n" ("Error Description") -> [_ w77]
      tunnel: [_ w76] -> w33
      frame False {
      }
      frame True {
        n185 = Format Into String(format string=w77, w79, w78) -> (resulting string=w76:string)  [unwired: 2 in, 1 out]
      }
    }
  }
  n186 = Unbundle By Name(w10) -> ("Major Vers"=w8:i32)
  n187 = Release Queue(queue=w30, error in (no error)=w28) -> (error out=w29:errorcluster)  [unwired: 1 in, 2 out]
  n188 = Concatenate Strings(w27) -> (w32:string)
  n189 = Greater?(x=w8, y=2) -> (0:w5:bool)
  n190 = Flattened String To Variant(4:w29, 6:w32, 7:w25) -> (0:→"Error Out":errorcluster, 3:→"Variant":variant)
  n191 = case shown="False" w5 {
    tunnel: w6 -> [w624 w628]
    tunnel: "Read/Write Anything File is newer than the code that handles it.  Data was read, but it may not be valid.\n" ("Error Description") -> [_ w627]
    tunnel: [w623 w626] -> w3
    tunnel: w1 -> [w622 w625]
    frame False {
      n192 = Concatenate Strings(w624, w622) -> (w623:string)
    }
    frame True {
      n193 = Concatenate Strings(w628, w627, w625) -> (w626:string)
    }
  }
  "Read Failures" <- w3
